vi "Error - unexpected response.vi"(8 "error in (no error)":errorcluster, 10 "Full Response":string) -> (0 "error out":errorcluster)   [LabVIEW 2017, in "FTP_UpgradeCSMF.lvlib" / "FTP.lvclass"]
uses:
  FTP.lvclass
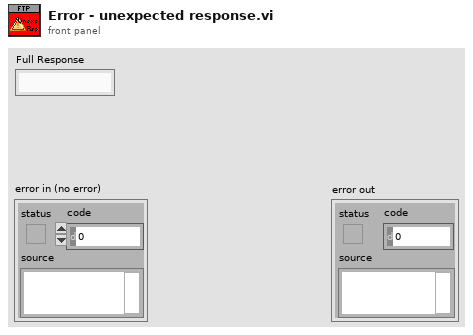
[diagram p1: front panel]
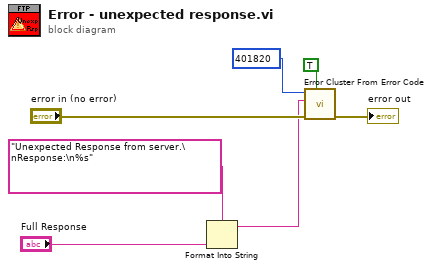
[diagram p0: block diagram]
diagram:
  n1 = Format Into String(format string="Unexpected Response from server.\nResponse:\n%s", "Full Response") -> (resulting string=w3:string)  [unwired: 2 in, 1 out]
  n2 = call <vilib>:"Error Cluster From Error Code.vi"("show call chain? (False)"=TRUE, "error in (no error)"="error in (no error)", "error message (\"\")"=w3, "error code (0)"=401820) -> ("error out"=→"error out":errorcluster)  [unwired: 5 in]
